vi "testErrorCodes.vi"(8 "error in (no error)":errorcluster, 11 "CoolerSerialCommand in":refnum<class "CoolerSerialCommand.lvclass">) -> (0 "error out":errorcluster, 3 "CoolerSerialCommand out":refnum<class "CoolerSerialCommand.lvclass">)   [LabVIEW 2016, in "CoolerSerialCommand.lvclass"]
uses:
  CoolerSerialCommand.lvclass
  typedefs/errorType.ctl
  <vilib>/addons/_JKI Toolkits/Caraya/classes/Test/Test.lvclass
  <vilib>/addons/_JKI Toolkits/Caraya/classes/Assert/Assert.lvclass
panel:
  in  "csv_error_list_file":path
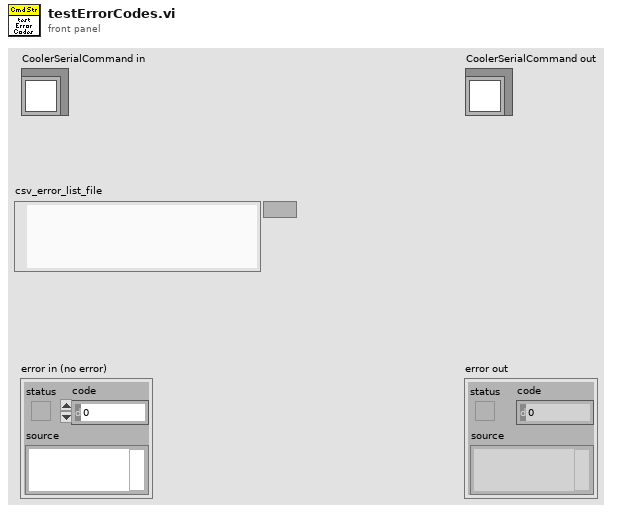
[diagram p1: front panel]
types:
  T1 = typedef "errorType.ctl" = cluster{"type":enum16{"AlarmStateLevel1", "AlarmStateLevel21", "AlarmStateLevel22", "WarningStateLevel1"}, "errorValue":u16}
  T2 = enum16{"AlarmStateLevel1", "AlarmStateLevel21", "AlarmStateLevel22", "WarningStateLevel1"}
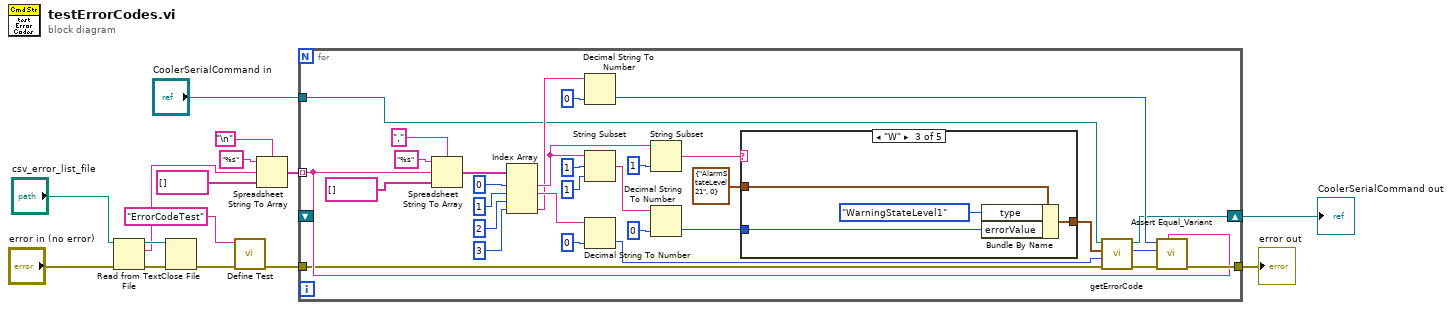
[diagram p0: block diagram]
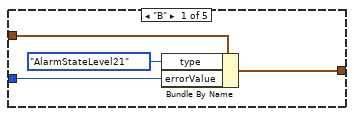
[diagram p2: hidden frame]
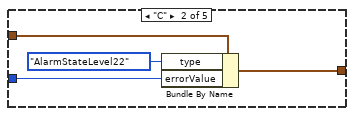
[diagram p3: hidden frame]
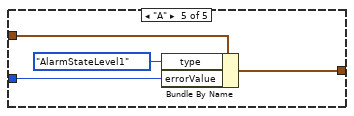
[diagram p5: hidden frame]
diagram:
  n1 = Read from Text File(file (use dialog)="csv_error_list_file", error in="error in (no error)") -> (refnum out=w12:refnum<file>, text=w8:string, error out=w11:errorcluster)  [unwired: 2 in, 1 out]
  n2 = Close File(refnum=w12, error in=w11) -> (error out=w10:errorcluster)  [unwired: 1 out]
  n3 = call <vilib>:"Define Test.vi"("error in (no error)"=w10, "Label (VI Title)"="ErrorCodeTest") -> ("error out"=w4:errorcluster)  [unwired: 9 in]
  n4 = Spreadsheet String To Array(delimiter (Tab)="\n", format string="%s", spreadsheet string=w8, array type (2D Dbl)=string[] []) -> (array=w5:string[])
  n5 = for {
    tunnel: w5 -> [w37] mode=indexing
    tunnel: w4 -> [w36]
    tunnel: [w38] -> w3
    tunnel: "CoolerSerialCommand in" -> [w17]
    shift-right: [w16] -> w1
    shift-left: _ -> [_]
    n6 = Spreadsheet String To Array(delimiter (Tab)=",", format string="%s", spreadsheet string=w37, array type (2D Dbl)=string[] []) -> (array=w43:string[])
    n7 = Index Array(array=w43, index #1=0 ("index"), index #2=1 ("index"), index #3=2 ("index"), index #4=3 ("index")) -> (element #1=w25:string, element #2=w23:string, element #4=w20:string)  [unwired: 1 out]
    n8 = Decimal String To Number(string=w20, default (0L)=u16 0 ("errorValue")) -> (number=w19:u16)  [unwired: 1 in, 1 out]
    n9 = String Subset(string=w25, offset (0)=1, length (rest)=1 ("length (rest)")) -> (substring=w28:string)
    n10 = Decimal String To Number(string=w23, default (0L)=u16 0 ("errorValue")) -> (number=w22:u16)  [unwired: 1 in, 1 out]
    n11 = String Subset(string=w25, length (rest)=1 ("length (rest)")) -> (substring=w32:string)  [unwired: 1 in]
    n12 = Decimal String To Number(string=w28, default (0L)=u16 0 ("errorValue")) -> (number=w26:u16)  [unwired: 1 in, 1 out]
    n13 = case shown="\"W\"" w32 {
      tunnel: T1 {"type"=enum."AlarmStateLevel21", "errorValue"=0} ("errorType") -> [w50 w53 w58 _ w62]
      tunnel: [w49 w54 w57 _ w61] -> w33
      tunnel: w26 -> [w47 w51 w55 _ w59]
      frame "B" {
        n14 = Bundle By Name(cluster=w50, "type"=T2."AlarmStateLevel21", "errorValue"=w47) -> (w49:T1)
      }
      frame "C" {
        n15 = Bundle By Name(cluster=w53, "type"=T2."AlarmStateLevel22", "errorValue"=w51) -> (w54:T1)
      }
      frame "W" {
        n16 = Bundle By Name(cluster=w58, "type"=T2."WarningStateLevel1", "errorValue"=w55) -> (w57:T1)
      }
      frame Default {
      }
      frame "A" {
        n17 = Bundle By Name(cluster=w62, "type"=T2."AlarmStateLevel1", "errorValue"=w59) -> (w61:T1)
      }
    }
    n18 = call "getErrorCode.vi"("error in (no error)"=w36, "code"=w22, "errorType"=w33, "CoolerSerialCommand in"=w17) -> ("error out"=w35:errorcluster, "errorCode"=w18:u16, "CoolerSerialCommand out"=w16:refnum<class "CoolerSerialCommand.lvclass">)  [unwired: 5 in]
    n19 = call <vilib>:"Assert Equal_Variant.vi"("Label"=w37, "error in (no error)"=w35, "Y"=w18, "X"=w19) -> ("error out"=w38:errorcluster)  [unwired: 7 in]
  }
  "error out" <- w3
  "CoolerSerialCommand out" <- w1
